vi "run script.vi"() -> ()   [LabVIEW 2016]
panel:
  out "BootFile error":errorcluster
  out "PreLoad error":errorcluster
  out "Run Script error":errorcluster
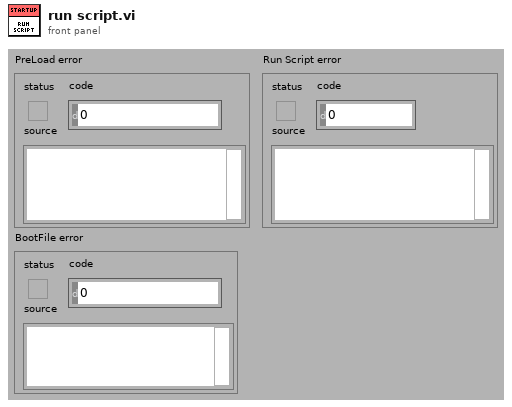
[diagram p1: front panel]
types:
  T1 = enum32{"Invalid", "Standard", "Closed", "Hidden", "Minimized", "Maximized"}
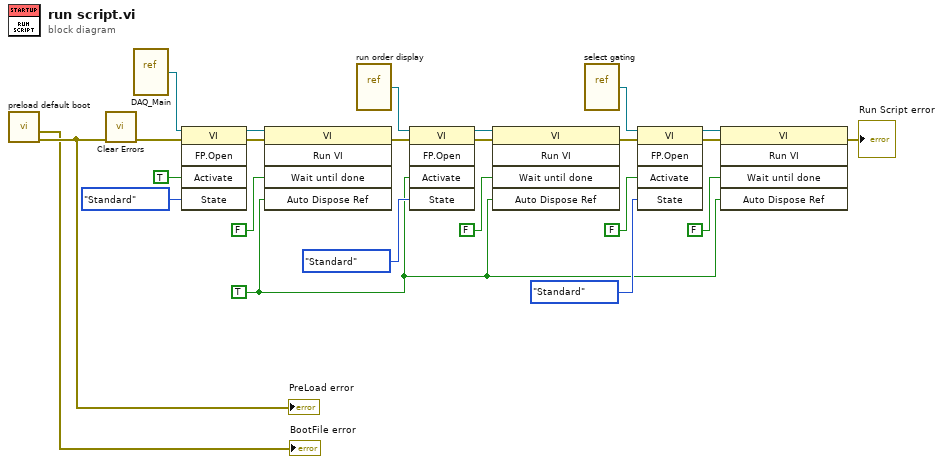
[diagram p0: block diagram]
diagram:
  w4 = TRUE ("Activate?")
  n1 = call "preload default boot.vi"() -> ("PreLoad error"=w21:errorcluster, "BootFile error"=→"BootFile error":errorcluster)  [unwired: 10 in]
  "PreLoad error" <- w21
  n2 = call <vilib>:"Clear Errors.vi"("error in (no error)"=w21) -> ("error out"=w2:errorcluster)  [unwired: 5 in, 1 out]
  n3 = vi-ref "DAQ_Main.vi"() -> (w24:refnum<vi>)
  n4 = invoke class="VI" method="FP.Open"(reference=w24, error in=w2, "Activate"=TRUE ("Activate?"), "State"=T1."Standard") -> (reference out=w18:refnum<vi>, error out=w20:errorcluster)  [unwired: 1 in, 3 out]
  n5 = invoke class="VI" method="Run VI"(reference=w18, error in=w20, "Wait until done"=FALSE ("Wait Until Done"), "Auto Dispose Ref"=w4) -> (error out=w12:errorcluster)  [unwired: 1 in, 4 out]
  n6 = vi-ref "run order display.vi"() -> (w13:refnum<vi>)
  n7 = invoke class="VI" method="FP.Open"(reference=w13, error in=w12, "Activate"=w4, "State"=T1."Standard") -> (reference out=w17:refnum<vi>, error out=w15:errorcluster)  [unwired: 1 in, 3 out]
  n8 = invoke class="VI" method="Run VI"(reference=w17, error in=w15, "Wait until done"=FALSE ("Wait Until Done"), "Auto Dispose Ref"=w4) -> (error out=w5:errorcluster)  [unwired: 1 in, 4 out]
  n9 = vi-ref "select gating.vi"() -> (w6:refnum<vi>)
  n10 = invoke class="VI" method="FP.Open"(reference=w6, error in=w5, "Activate"=FALSE ("Activate?"), "State"=T1."Standard") -> (reference out=w7:refnum<vi>, error out=w9:errorcluster)  [unwired: 1 in, 3 out]
  n11 = invoke class="VI" method="Run VI"(reference=w7, error in=w9, "Wait until done"=FALSE ("Wait Until Done"), "Auto Dispose Ref"=w4) -> (error out=→"Run Script error":errorcluster)  [unwired: 1 in, 4 out]
